vi "LPF for CF.vi"(10 "Numeric":dbl) -> (2 "Numeric 2":dbl)   [LabVIEW 2011]
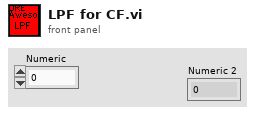
[diagram p1: front panel]
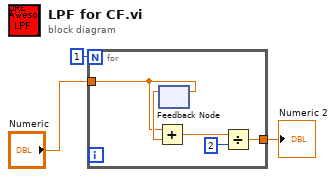
[diagram p0: block diagram]
diagram:
  n1 = for {
    N: 1 -> [_]
    tunnel: [w7] -> w2
    tunnel: "Numeric" -> [w4]
    n2 = feedback #1() -> (w5:dbl)  [unwired: 1 in]
    n3 = Add(x=w4, y=w5) -> (x+y=w6:dbl)
    n4 = feedback-in #1(w4) -> ()
    n5 = Divide(x=w6, y=2) -> (x/y=w7:dbl)
  }
  "Numeric 2" <- w2
